vi "Complex Polynomial Roots.vi"(0 "Polynomial":cdb[](array[numeric]) format="%0.2f") -> (1 "Polynomial Roots":cdb[](array[numeric]) format="%0.2f", 2 "error":i32)   [LabVIEW 2020, in "NI_AALPro.lvlib"]
doc: "Finds the complex roots of a complex polynomial."
uses:
  NI_AALPro.lvlib
  <resource>/lvanlys.dll
panel:
  # "Complex Polynomial Roots"
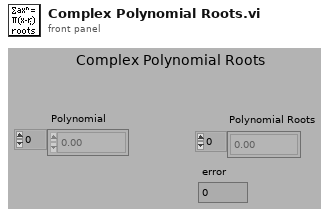
[diagram p1: front panel]
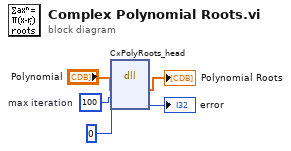
[diagram p0: block diagram]
diagram:
  w4 = 100  # max iteration
  n1 = dll-call lib="C:/Program Files (x86)/National Instruments/LabVIEW 2020/resource/lvanlys.*" fn="CxPolyRoots_head"("Polynomial"="Polynomial", "max iteration"=w4, 0) -> ("Polynomial"=→"Polynomial Roots":cdb[], →"error":i32)  [unwired: 5 in, 2 out]
